vi "Get_GridParams (SubVI).vi"(8 "error in (no error)":errorcluster, 9 "Grid Settings":T1={"type"=1, "type order"=1, "X pixel"=0.0, "Y pixel"=0.0, "Grid_Parms"={"center X (m)"=0.0, "center Y (m)"=0.0, "width (m)"=0.0, "height (m)"=0.0, "angle (deg)"=0.0}} {"type order" items=["Line", "Grid"]; "type" items=["Line", "Grid"]}, 11 "Application in":refnum<vi>) -> (0 "error out":errorcluster, 1 "Grid Settings":T1, 2 "total Points":i32=2500, 3 "Application out":refnum<vi>)   [LabVIEW 2014]
uses:
  <userlib>/Nanonis Prog Interface V5/Scan/Grid/GridPatternGet.vi
  <userlib>/Nanonis Prog Interface V5/Scan/Grid/CloudPatternGet.vi
  <userlib>/Nanonis Prog Interface V5/Scan/Grid/LinePatternGet.vi
  <userlib>/Nanonis Prog Interface V5/Nanonis Prog Interface.lvlib
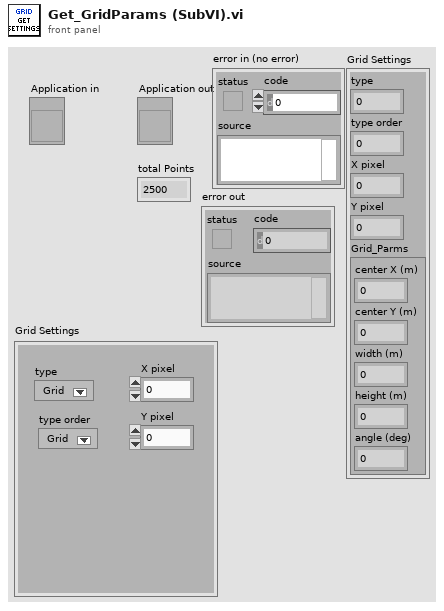
[diagram p1: front panel]
types:
  T1 = cluster{"type":u16, "type order":u16, "X pixel":dbl, "Y pixel":dbl, "Grid_Parms":cluster{"center X (m)":sgl, "center Y (m)":sgl, "width (m)":sgl, "height (m)":sgl, "angle (deg)":sgl}}
  T2 = cluster{"center X (m)":sgl, "center Y (m)":sgl, "width (m)":sgl, "height (m)":sgl, "angle (deg)":sgl}
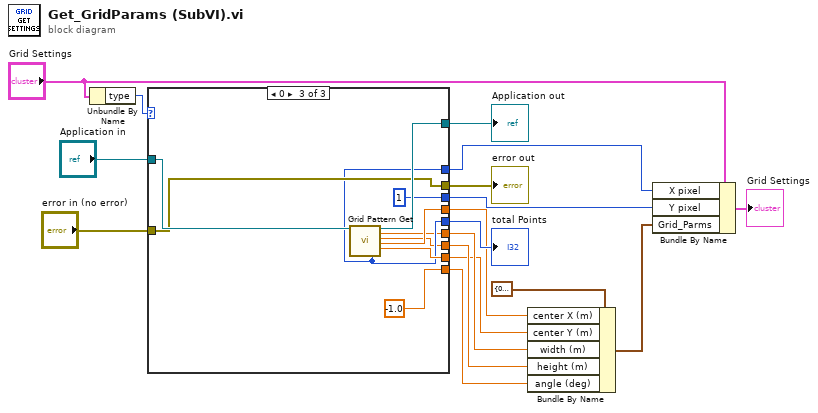
[diagram p0: block diagram]
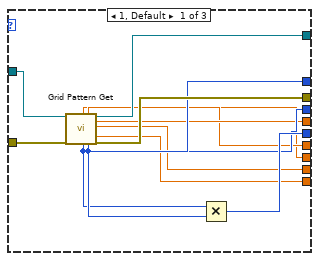
[diagram p2: hidden frame]
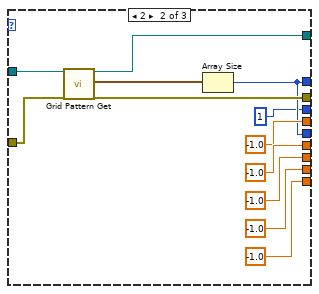
[diagram p3: hidden frame]
diagram:
  n1 = Unbundle By Name("Grid Settings") -> ("type"=w8:u16)
  n2 = case shown="0" w8 {
    tunnel: [w29 w40 w51] -> w17
    tunnel: [w28 w31 w45] -> w15
    tunnel: "Application in" -> [w27 w41 w50]
    tunnel: "error in (no error)" -> [w26 w38 w49]
    tunnel: [w25 w39 w49] -> w13
    tunnel: [w19 sgl -1.0 ("Start X1 (m)") w43] -> w3
    tunnel: [w21 sgl -1.0 ("End Y2 (m)") w47] -> w1
    tunnel: [w22 sgl -1.0 ("End X2 (m)") w48] -> w2
    tunnel: [w18 sgl -1.0 ("Angle (°)") sgl -1.0 ("Angle (°)")] -> w4
    tunnel: [w20 sgl -1.0 ("Start Y1 (m)") w42] -> w5
    tunnel: [w24 w31 w45] -> w7
    tunnel: [w23 1 ("Points Y") 1 ("Points Y")] -> w6
    frame 1, Default {
      n3 = call-poly <userlib>:"Grid Pattern Get.vi"("Application ref in"=w27, "error in (no error)"=w26) -> ("Height (m)"=w19:sgl, "Points Y"=w23:i32, "Width (m)"=w20:sgl, "Points X"=w24:i32, "Application ref out"=w29:refnum<vi>, "Center Xc (m)"=w22:sgl, "Center Yc (m)"=w21:sgl, "Angle (°)"=w18:sgl, "error out"=w25:errorcluster)  [unwired: 9 in]
      n4 = Multiply(x=w23, y=w24) -> (x*y=w28:i32)
    }
    frame 2 {
      n5 = call-poly <userlib>:"Grid Pattern Get.vi"("Application ref in"=w41, "error in (no error)"=w38) -> ("Application ref out"=w40:refnum<vi>, "Cloud data"=w37:cluster{"X":sgl, "Y":sgl}[], "error out"=w39:errorcluster)  [unwired: 15 in]
      n6 = Array Size(array=w37) -> (size(s)=w31:i32)
    }
    frame 0 {
      n7 = call-poly <userlib>:"Grid Pattern Get.vi"("Application ref in"=w50) -> ("Points"=w45:i32, "Application ref out"=w51:refnum<vi>, "Start X1 (m)"=w42:sgl, "Start Y1 (m)"=w43:sgl, "End X2 (m)"=w48:sgl, "End Y2 (m)"=w47:sgl)  [unwired: 12 in, 1 out]
    }
  }
  "total Points" <- w15
  "Application out" <- w17
  "error out" <- w13
  n8 = Bundle By Name(cluster=T2 {"center X (m)"=0.0, "center Y (m)"=0.0, "width (m)"=0.0, "height (m)"=0.0, "angle (deg)"=0.0} ("Grid param"), "center X (m)"=w2, "center Y (m)"=w1, "width (m)"=w5, "height (m)"=w3, "angle (deg)"=w4) -> (w11:T2)
  n9 = Bundle By Name(cluster="Grid Settings", "X pixel"=w7, "Y pixel"=w6, "Grid_Parms"=w11) -> (→"Grid Settings":T1)
